vi "Ultrasonic.vi"() -> ()   [LabVIEW 2025]
doc: "This example shows how to use an SRF04 Ultra-Sonic Ranger.\n\nIt will display the distance from the sensor in inches or mm.\n\nThe SRF04 has a range from 3 inches to 120 inches. It uses two digital lines. For this example the sensor Ping is connected to S of digital I/O 6, and the sensor Echo is connected to S of digital I/O 7. The sensor ground should be connected to the ground pin of either digital channel, and the sensor +5V should be connected to the V pin of either digital channel.\n\nTiming considerations. The SRF04 works by sending it a 10us ping. This causes an 8 cycle sonic burst from the sensor. The echo pulse ranges from 100us to 18ms, but can be as long as 36ms if no object is detected. Finally a 10ms delay is needed from the end of the echo to the next ping. The loop rate of this example is 10 times per second. In practice, maximum loop rates could be 30 times per second.\n\nThis example expects a USB cable connected from your development PC to the Type B USB Jack (next to the power input) on the roboRIO.\n\nThis example expects the Driver Station to be running."
uses:
  <vilib>/Rock Robotics/WPI/Ultrasonic/WPI_UltrasonicRangeUnits.ctl
  <vilib>/Rock Robotics/SystemInterfaces/DIO/FPGA_DIOChannel.ctl
  <vilib>/Rock Robotics/WPI/Ultrasonic/WPI_SonarSRF04DigitalOpen.vi
  <vilib>/Rock Robotics/WPI/Ultrasonic/WPI_SonarSRF04DigitalGetRange.vi
  <vilib>/Rock Robotics/WPI/Ultrasonic/WPI_SonarSRF04DigitalClose.vi
panel:
  out "units":string="inches"
  in  "Ping DIO Channel":T1=enum."DIO 6"
  in  "Echo DIO Channel":T1=enum."DIO 7"
  out "distance":dbl(slide)=60.0 scale=0.0..120.0 scale format="%#.3g"
  in  "pingtime (Sec)":sgl=1e-05
  in  "Range Units":T2
  in  "stop":bool
  # "Set these inputs before running."
  # "These can be set while running."
  # "SRF04"
  # "Output information."
  # "This shows wiring for an SRF04 ultrasonic sensor."
  # "SRF04\n+5V (red)---------\nEcho (white)-----\nPing (white)------\nGnd (black)------"
  # "roboRIO\nDIO-6  V\nDIO-7  S\nDIO-6  S\nDIO-6"
  # "SRF04"
  # "+5V"
  # "Echo"
  # "Ping"
  # "Gnd"
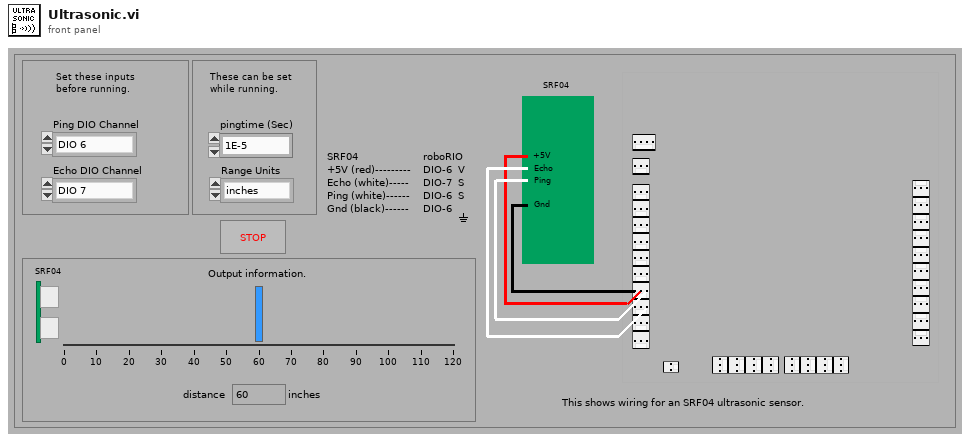
[diagram p1: front panel]
types:
  T1 = typedef "FPGA_DIOChannel.ctl" = enum8{"DIO 0", "DIO 1", "DIO 2", "DIO 3", "DIO 4", "DIO 5", "DIO 6", "DIO 7", "DIO 8", "DIO 9", "DIO MXP 0", "DIO MXP 1", "DIO MXP 2", "DIO MXP 3", "DIO MXP 4", "DIO MXP 5", "DIO MXP 6", "DIO MXP 7", "DIO MXP 8", "DIO MXP 9", "DIO MXP 10", "DIO MXP 11", "DIO MXP 12", "DIO MXP 13", "DIO MXP 14", "DIO MXP 15", "SPI Port CS1", "SPI Port CS2", "SPI Port CS3", "SPI Port MISO", "SPI Port MOSI", "Invalid"}
  T2 = typedef "WPI_UltrasonicRangeUnits.ctl" = enum16{"inches", "mm"}
  T3 = typedef "WPI_UltrasonicDeviceRef.ctl" = cluster{"DevStatus":errorcluster, "Ping Channel":T1, "Echo Channel":T1, "CntIndex":T4}
  T4 = typedef "FPGA_CounterCtrSystemIndex.ctl" = enum8{"Ctr 0", "Ctr 1", "Ctr 2", "Ctr 3", "Ctr 4", "Ctr 5", "Ctr 6", "Ctr 7", "Invalid"}
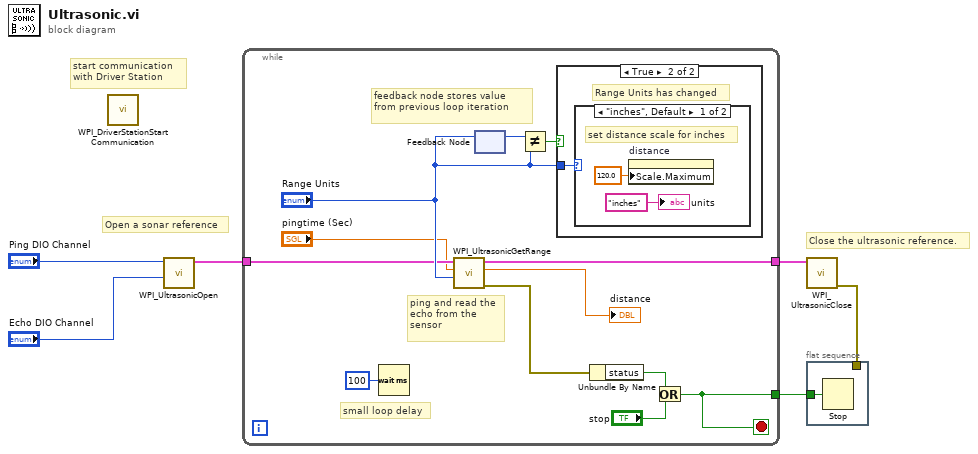
[diagram p0: block diagram]
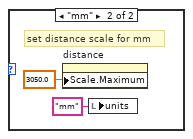
[diagram p3: hidden frame]
diagram:
  # "start communication with Driver Station"
  # "Close the ultrasonic reference."
  # "Open a sonar reference"
  n1 = call <vilib>:"WPI_DriverStationStart Communication.vi"() -> ()  [unwired: 3 in, 9 out]
  n2 = call-poly <vilib>:"WPI_UltrasonicOpen.vi"("Echo DIO Channel"="Echo DIO Channel", "Ping DIO Channel"="Ping DIO Channel") -> ("UltrasonicDevRef"=w3:T3)  [unwired: 8 in, 1 out]
  n3 = while {
    tunnel: w3 -> [w8]
    tunnel: [w18] -> w4
    tunnel: [w9] -> w2
    stop <- w9 stop-if-true
    # "feedback node stores value from previous loop iteration"
    # "ping and read the echo from the sensor"
    # "small loop delay"
    n4 = Wait (ms)(milliseconds to wait=u32 100) -> ()  [unwired: 1 out]
    n5 = call-poly <vilib>:"WPI_UltrasonicGetRange.vi"("Range Units"="Range Units", "ping time (s)"="pingtime (Sec)", "UltrasonicDevRef"=w8) -> ("error out"=w17:errorcluster, "Distance"=→"distance":dbl, "UltrasonicDevRef"=w18:T3)  [unwired: 6 in]
    n6 = feedback-in #1("Range Units") -> ()
    n7 = feedback #1() -> (w12:T2)  [unwired: 1 out]
    n8 = Not Equal?(x=w12, y="Range Units") -> (x != y?=w11:bool)
    n9 = case shown="True" w11 {
      tunnel: "Range Units" -> [_ w19]
      frame False {
        # "Range Units has not changed"
      }
      frame True {
        # "Range Units has changed"
        n10 = case shown="\"inches\", Default" w19 {
          frame "inches", Default {
            # "set distance scale for inches"
            n11 = property on="distance" class="Slide (strict)"("Scale.Maximum"=120.0 ("Scale.Range:Maximum")) -> ()  [unwired: 2 in, 2 out]
            "units" <- "inches" ("units")
          }
          frame "mm" {
            # "set distance scale for mm"
            n12 = property on="distance" class="Slide (strict)"("Scale.Maximum"=3050.0 ("Scale.Range:Maximum")) -> ()  [unwired: 2 in, 2 out]
            n13 = local write "units"("mm" ("units")) -> ()
          }
        }
      }
    }
    n14 = Unbundle By Name(w17) -> ("status"=w15:bool)
    n15 = Or(x=w15, y="stop") -> (x .or. y?=w9:bool)
  }
  n16 = call-poly <vilib>:"WPI_UltrasonicClose.vi"("UltrasonicDevRef"=w4) -> ("error out"=w1:errorcluster)  [unwired: 10 in]
  n17 = flat-sequence {
    tunnel: w2 -> [w24]
    tunnel: w1 -> [_]
    frame #0 {
      n18 = Stop(stop? (T)=w24) -> ()
    }
  }
